vi "Get VI Breakpoints.vi"(8 "error in":errorcluster, 10 "Class Name":T3, 11 "VI Reference in":refnum<vi>) -> (0 "error out":errorcluster, 2 "Breakpoints":T1[](array[typedef]), 3 "VI Reference out":refnum<vi>)   [LabVIEW 2020]
doc: "This VI retrieves breakpoint information for the specified class in the active VI."
uses:
  Type Definitions/Class Name--enum.ctl
  Type Definitions/Breakpoint--cluster.ctl
  <vilib>/Utility/miscctls.llb/LVBreakpointStatusEnum.ctl
  <vilib>/Utility/traverseref.llb/TRef TravTarget.ctl
  <vilib>/Utility/traverseref.llb/VI Scripting - Traverse.lvlib
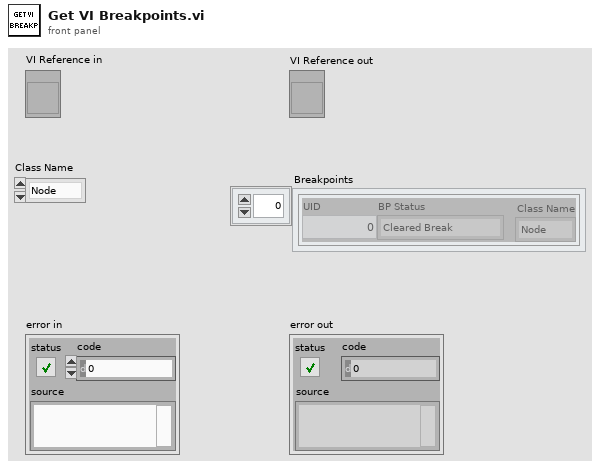
[diagram p1: front panel]
types:
  T1 = typedef "Breakpoint--cluster.ctl" = cluster{"UID":i32, "BP Status":T2, "Class Name":T3}
  T2 = typedef "LVBreakpointStatusEnum.ctl" = enum8{"Cleared Break", "Enabled Break", "Disabled Break"}
  T3 = typedef "Class Name--enum.ctl" = enum16{"Node", "Wire"}
  T4 = typedef "TRef TravTarget.ctl" = enum16{"FP", "BD", "Other"}
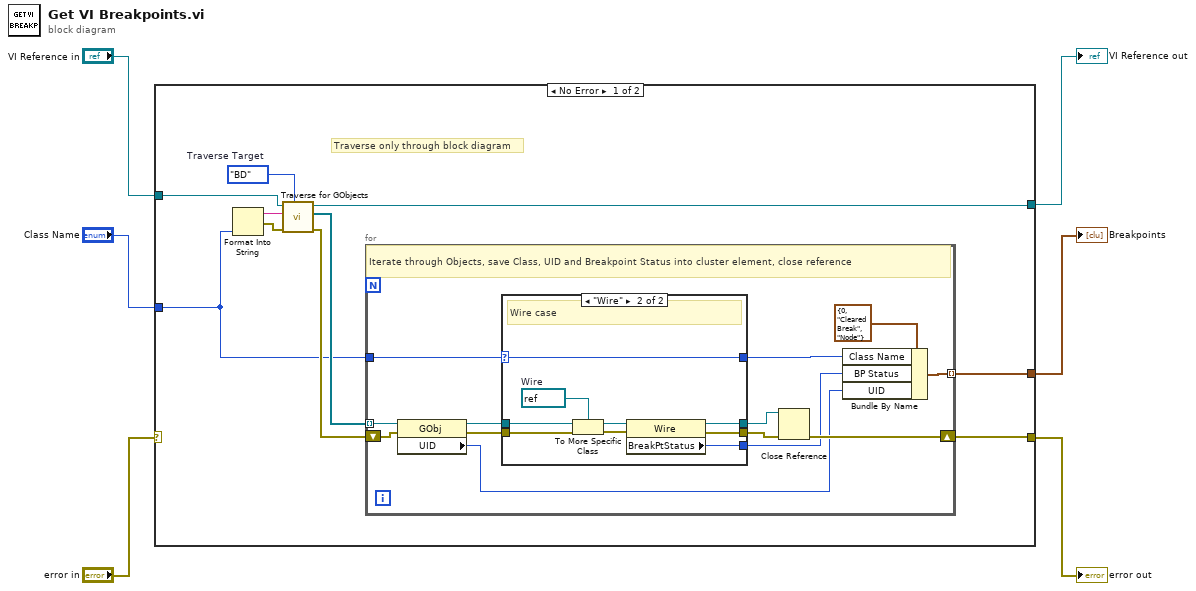
[diagram p0: block diagram]
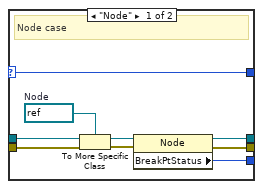
[diagram p2: hidden frame]
diagram:
  n1 = case shown="No Error" "error in" {
    selector: "error in" -> [_ w48]
    tunnel: "VI Reference in" -> [w13 _]
    tunnel: "Class Name" -> [w9 _]
    tunnel: [w8 _] -> w1
    tunnel: [w14 w48] -> w5
    tunnel: [w7 _] -> w2
    frame No Error {
      w12 = TRef_TravTarget."BD"  # Traverse Target
      # "Traverse only through block diagram"
      n2 = Format Into String(w9) -> (resulting string=w10:string, error out=w15:errorcluster)  [unwired: 3 in]
      n3 = call <vilib>:"Traverse for GObjects.vi"("Traverse Target"=w12, "error in (no error)"=w15, "Class Name"=w10, "VI Refnum"=w13) -> ("error out"=w16:errorcluster, "References"=w11:refnum<vi>[], "dup VI Refnum"=w8:refnum<vi>)  [unwired: 4 in, 1 out]
      n4 = for {
        tunnel: w11 -> [w25] mode=indexing
        shift-right: [w26] -> w14
        shift-left: w16 -> [w29]
        tunnel: [w20] -> w7 mode=indexing
        tunnel: w9 -> [w18]
        # "Iterate through Objects, save Class, UID and Breakpoint Status into cluster element, close reference"
        n5 = property class="GObj"(reference=w25, error in=w29) -> (reference out=w24:refnum<vi>, error out=w28:errorcluster, "UID"=w17:i32)
        n6 = case shown="\"Wire\"" w18 {
          selector: w18 -> [w30 w40]
          tunnel: w24 -> [w35 w44]
          tunnel: w28 -> [w38 w47]
          tunnel: [w36 w45] -> w27
          tunnel: [w33 w43] -> w23
          tunnel: [w32 w42] -> w21
          tunnel: [w30 w40] -> w19
          frame "Node" {
            w31 = refnum<vi> refnum  # Node
            # "Node case"
            n7 = To More Specific Class(target class=w31, reference=w35, error in=w38) -> (specific class reference=w34:refnum<vi>, error out=w37:errorcluster)
            n8 = property class="Node"(reference=w34, error in=w37) -> (reference out=w33:refnum<vi>, error out=w36:errorcluster, "BreakPtStatus"=w32:T2)
          }
          frame "Wire" {
            w41 = refnum<vi> refnum  # Wire
            # "Wire case"
            n9 = To More Specific Class(target class=w41, reference=w44, error in=w47) -> (specific class reference=w39:refnum<vi>, error out=w46:errorcluster)
            n10 = property class="Wire"(reference=w39, error in=w46) -> (reference out=w43:refnum<vi>, error out=w45:errorcluster, "BreakPtStatus"=w42:T2)
          }
        }
        n11 = Close Reference(reference=w23, error in (no error)=w27) -> (error out=w26:errorcluster)
        n12 = Bundle By Name(cluster=T1 {"UID"=0, "BP Status"=enum."Cleared Break", "Class Name"=enum."Node"} ("Breakpoint"), "Class Name"=w19, "BP Status"=w21, "UID"=w17) -> (w20:T1)
      }
    }
    frame Error {
      # "Pass error without further action"
    }
  }
  "VI Reference out" <- w1
  "error out" <- w5
  "Breakpoints" <- w2
